vi "Close.vi"(8 "error in (no error)":errorcluster, 11 "LINX I2C in":refnum<class "LINX I2C.lvclass">) -> (0 "error out":errorcluster, 3 "LINX I2C out":refnum<class "LINX I2C.lvclass">)   [LabVIEW 2020, in "LINX I2C.lvclass"]
uses:
  LINX I2C.lvclass
  LINX I2C.lvclass/LINX I2C.ctl
  <vilib>/MakerHub/LINX/LMH-LINX.lvlib
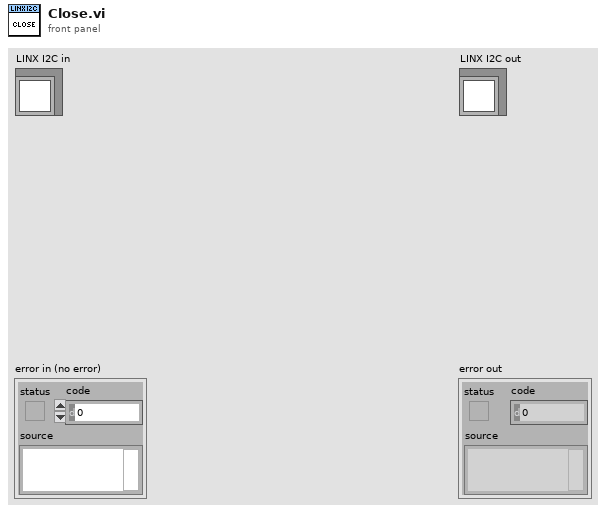
[diagram p1: front panel]
types:
  T1 = typedef "LMH-LINX.lvlib/LINX Ref.ctl" = cluster{"IO":T2, "Interface":T3, "LINX Device Config":T4}
  T2 = typedef "LMH-LINX.lvlib/Platform.ctl" = enum16{"Remote", "Local"}
  T3 = typedef "LMH-LINX.lvlib/Interface.ctl" = enum16{"Serial", "TCP"}
  T4 = typedef "LMH-LINX.lvlib/Device.lvlib/LINX Device Config.ctl" = cluster{"Interface":T3, "COM Port":refnum<visa-resource-name>, "TCP Configuration":T5, "Device Family":u8, "Device ID":u8, "Device Name":string, "TCP Ref":refnum<k5>, "Channels":T6}
  T5 = typedef "LMH-LINX.lvlib/Device.lvlib/TCP Config.ctl" = cluster{"IP Address":string, "Port":u16}
  T6 = typedef "LMH-LINX.lvlib/Channels.ctl" = cluster{"DI":u8[], "DO":u8[], "AI":u8[], "AO":u8[], "PWM":u8[], "QE":u8[], "UART":u8[], "I2C 2":u8[], "SPI":u8[], "CAN":u8[], "Servo":u8[], "AI Ref (V)":dbl, "AI Resolution (Bits)":u8, "AO Ref (V)":dbl, "AO Resolution (Bits)":u8}
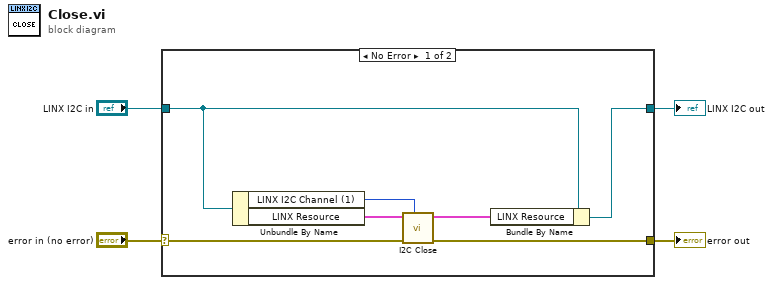
[diagram p0: block diagram]
diagram:
  n1 = case shown="No Error" "error in (no error)" {
    selector: "error in (no error)" -> [w8 w13]
    tunnel: [w6 w13] -> w3
    tunnel: [w10 w12] -> w1
    tunnel: "LINX I2C in" -> [w11 w12]
    frame No Error {
      n2 = Unbundle By Name(w11) -> ("LINX I2C Channel (1)"=w5:u8, "LINX Resource"=w9:T1)
      n3 = call <vilib>:"I2C Close.vi"("I2C Channel (0)"=w5, "Error In"=w8, "LINX Resource"=w9) -> ("Error Out"=w6:errorcluster, "LINX Resource"=w7:T1)  [unwired: 7 in]
      n4 = Bundle By Name(cluster=w11, "LINX Resource"=w7) -> (w10:refnum<class "LINX I2C.lvclass">)
    }
    frame Error {
    }
  }
  "error out" <- w3
  "LINX I2C out" <- w1
